vi "GPIB write rf ramp linear up for SG380.vi"(3 "calculate":bool, 5 "do it!":bool, 6 "debug":bool, 7 "time step (ms)":dbl=50.0 format="%.2f", 8 "Sweeps":T1(array[cluster])=[{"Enable MW"=FALSE, "MW End freq"="6810", "MW Tau (s)"="7", "MW Amplitude (dB)"="-3", "MW Comments"=""}, {"Enable MW"=FALSE, "MW End freq"="6820", "MW Tau (s)"="7", "MW Amplitude (dB)"="-5", "MW Comments"=""}, {"Enable MW"=FALSE, "MW End freq"="6830", "MW Tau (s)"="5", "MW Amplitude (dB)"="-5", "MW Comments"=""}, {"Enable MW"=FALSE, "MW End freq"="6832", "MW Tau (s)"="1", "MW Amplitude (dB)"="-7", "MW Comments"=""}, {"Enable MW"=FALSE, "MW End freq"="6833.22", "MW Tau (s)"="1", "MW Amplitude (dB)"="-8", "MW Comments"=""}], 9 "start freq (MHz)":string="6700.00", 10 "start time (sec)":string="1.000") -> (0 "start freq 2":dbl=6700.0, 1 "start time 2":dbl=1.0, 2 "calc'd time":dbl=1.0 format="%.3f", 4 "timing check":dbl=6.484375 format="%.3f")   [LabVIEW 2017]
uses:
  <vilib>/Utility/file.llb/Write Delimited Spreadsheet (DBL).vi
panel:
  out "Numeric":i32
  out "error out 3":errorcluster={"status"=TRUE, "code"=2, "source"="GPIB Write in rf ramp newest.vi"}
  in  "write":string="FREQ 6 MHz"
  in  "TEST":bool
  in  "GPIB address":string="27"
  out "error out 2":errorcluster={"status"=TRUE, "code"=7, "source"="GPIB Write in GPIB write rf ramp linear up for SG380.vi->host 1st.vi"}
  out "New sweeps array":dbl[][](array[numeric])
  out "error out":errorcluster
  out "XY Graph":cluster{"times":dbl[], "freqs":dbl[]}(graph)
  out "freqs":dbl[](array[numeric]) format="%.2f"
  out "times":dbl[](array[numeric])=[6700.0] format="%.2f"
  out "Path":path=path "C:/Debbie/experiment stuff/B231/13 Experiment Control/C code files/rf Ramp (2003 July 18)/rf ramp debug.txt"
  out "clock start":dbl=3608801724.173161 format="%.2f"
  out "freqs":dbl[](array[numeric])=[6700.0] format="%.2f"
  out "nramps":i32
  # "enable     f (MHz)           tau (sec)             ampl (dBm)                    notes"
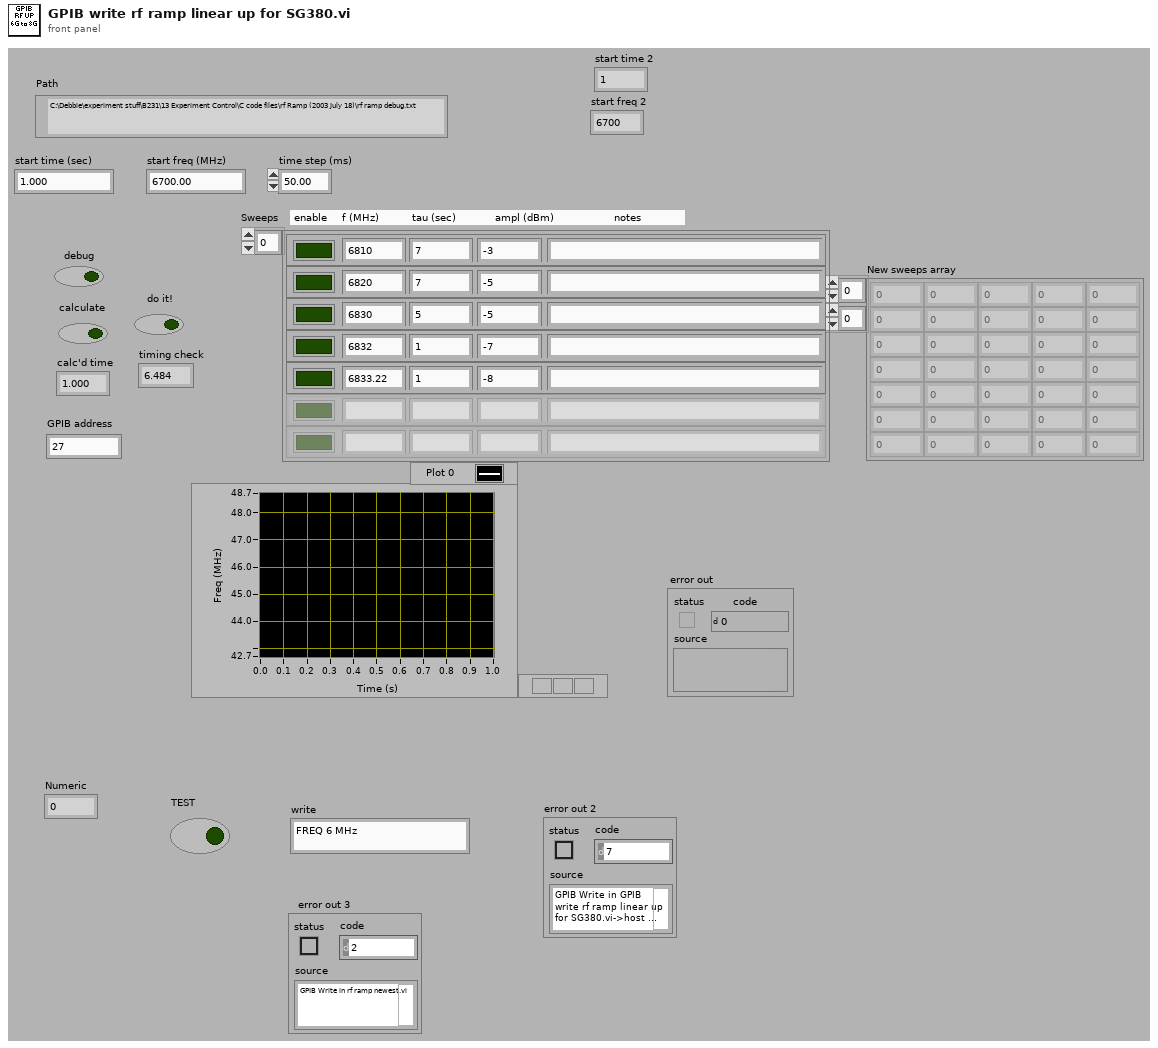
[diagram p1: front panel]
types:
  T1 = cluster{"Enable MW":bool, "MW End freq":string, "MW Tau (s)":string, "MW Amplitude (dB)":string, "MW Comments":string}[]
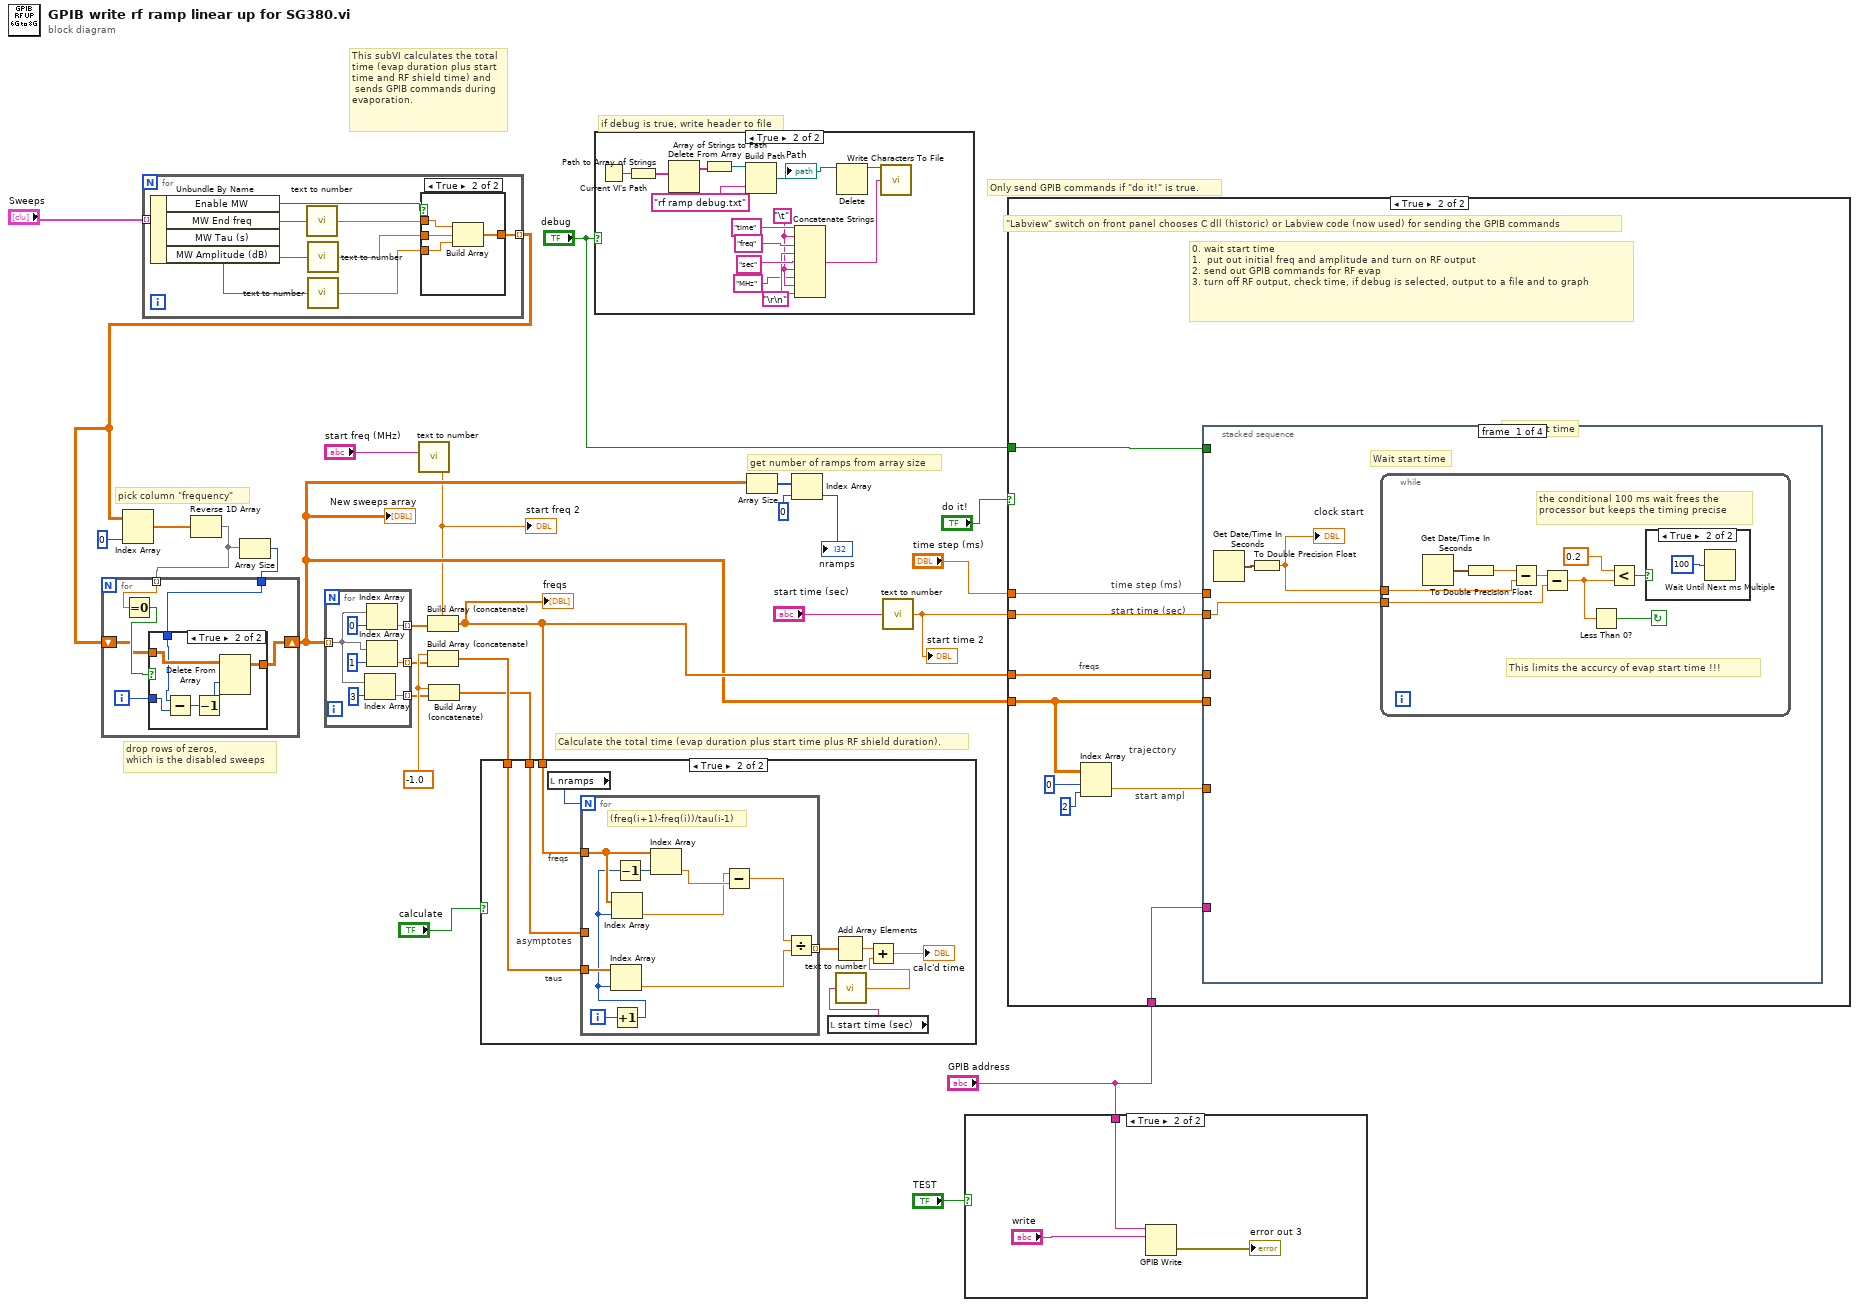
[diagram p0: block diagram]
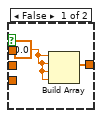
[diagram p4: hidden frame]
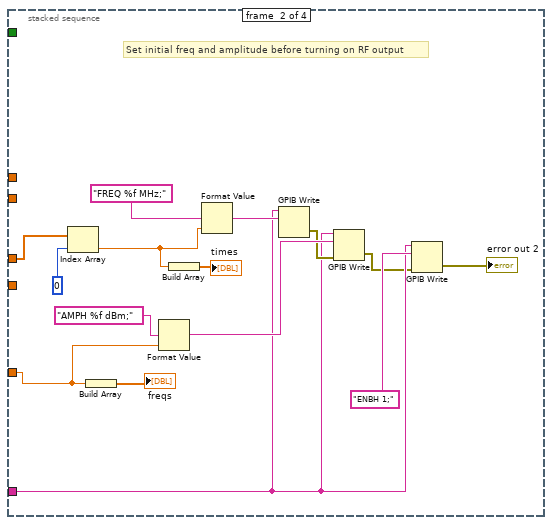
[diagram p7: hidden frame]
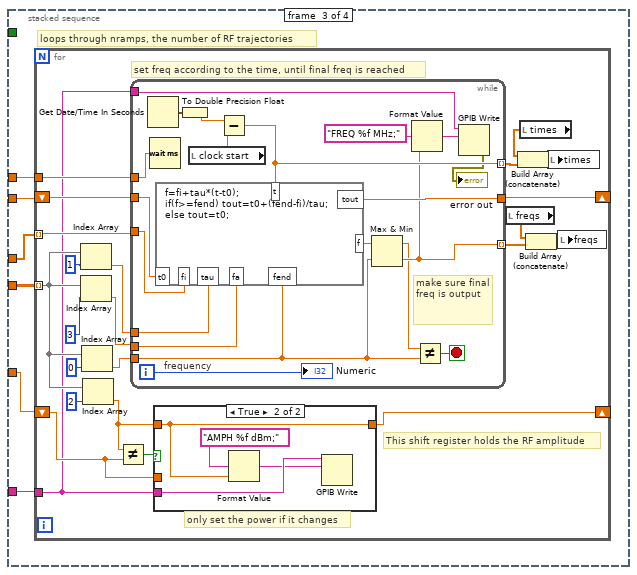
[diagram p8: hidden frame]
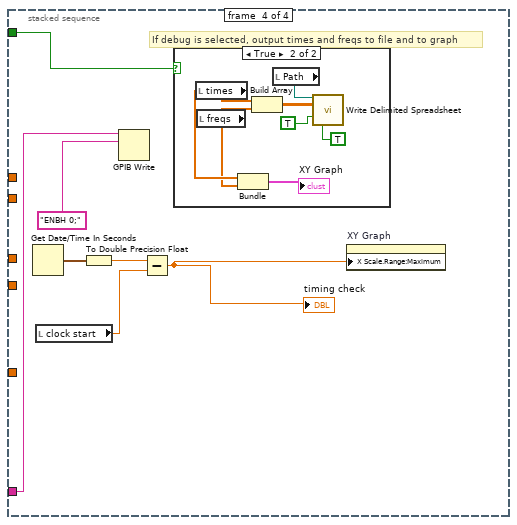
[diagram p10: hidden frame]
diagram:
  w18 = -1.0
  # "drop rows of zeros,\nwhich is the disabled sweeps"
  # "pick column \"frequency\""
  # "Only send GPIB commands if \"do it!\" is true."
  # "if debug is true, write header to file"
  # "This subVI calculates the total time (evap duration plus start time and RF shield time) and\n sends GPIB commands during evaporation."
  # "Calculate the total time (evap duration plus start time plus RF shield duration)."
  # "get number of ramps from array size"
  n1 = for {
    tunnel: "Sweeps" -> [w36] mode=indexing
    tunnel: [w34] -> w15 mode=indexing
    n2 = Unbundle By Name(w36) -> ("Enable MW"=w35:bool, "MW End freq"=w33:string, "MW Tau (s)"=w31:string, "MW Amplitude (dB)"=w30:string)
    n3 = call "text to number.vi"("text"=w33) -> ("number"=w32:dbl)
    n4 = call "text to number.vi"("text"=w31) -> ("number"=w29:dbl)
    n5 = call "text to number.vi"("text"=w30) -> ("number"=w28:dbl)
    n6 = case shown="True" w35 {
      tunnel: w32 -> [_ w42]
      tunnel: w29 -> [_ w41]
      tunnel: w28 -> [_ w40]
      tunnel: [w38 w39] -> w34
      frame False {
        w37 = 0.0 ("element")
        n7 = Build Array(w37, w37, w37, w37) -> (w38:dbl[])
      }
      frame True {
        n8 = Build Array(w42, w41, w40) -> (w39:dbl[])
      }
    }
  }
  n9 = Index Array(array=w15, index (col)=i8 0 ("Column #")) -> (element=w8:dbl[])  [unwired: 1 in]
  n10 = Reverse 1D Array(array=w8) -> (reversed array=w7:dbl[])
  n11 = Array Size(array=w7) -> (size(s)=w6:i32)
  n12 = for {
    tunnel: w7 -> [w48] mode=indexing
    shift-right: [w45] -> w9
    shift-left: w15 -> [w46]
    tunnel: w6 -> [w44]
    i -> [w43]
    n13 = Equal To 0?(x=w48) -> (x = 0?=w47:bool)
    n14 = case shown="True" w47 {
      tunnel: w46 -> [w49 w55]
      tunnel: w43 -> [_ w52]
      tunnel: [w49 w54] -> w45
      tunnel: w44 -> [_ w53]
      frame False {
      }
      frame True {
        n15 = Subtract(x=w53, y=w52) -> (x-y=w50:i32)
        n16 = Decrement(x=w50) -> (x-1=w51:i32)
        n17 = Delete From Array(array=w55, index (row)=w51) -> (array with subset deleted=w54:dbl[][])  [unwired: 2 in, 1 out]
      }
    }
  }
  "New sweeps array" <- w9
  n18 = for {
    tunnel: [w60] -> w12 mode=indexing
    tunnel: [w59] -> w11 mode=indexing
    tunnel: [w57] -> w10 mode=indexing
    tunnel: w9 -> [w56] mode=indexing
    n19 = Index Array(array=w56, index=3 ("Index")) -> (element=w57:dbl)
    n20 = Index Array(array=w56, index=0 ("Index")) -> (element=w60:dbl)
    n21 = Index Array(array=w56, index=1 ("Index")) -> (element=w59:dbl)
  }
  n22 = call "text to number.vi"("text"="start freq (MHz)") -> ("number"=w3:dbl)
  "start freq 2" <- w3
  n23 = Build Array (concatenate)(w3, w12) -> (w22:dbl[])
  "freqs" <- w22
  n24 = Build Array (concatenate)(w18, w11) -> (w21:dbl[])
  n25 = Build Array (concatenate)(w18, w10) -> (w20:dbl[])
  n26 = case shown="True" "calculate" {
    tunnel: w22 -> [_ w70]
    tunnel: w21 -> [_ w69]
    tunnel: w20 -> [_ w66]
    frame False {
    }
    frame True {
      # "taus"
      # "asymptotes"
      # "freqs"
      n27 = local read "nramps"() -> (w71:i32)
      n28 = for {
        N: w71 -> [_]
        tunnel: w70 -> [w79]
        tunnel: w69 -> [w81]
        tunnel: [w76] -> w68 mode=indexing
        tunnel: w66 -> [_]
        i -> [w78]
        # "(freq(i+1)-freq(i))/tau(i-1)"
        n29 = Increment(x=w78) -> (x+1=w77:i32)
        n30 = Index Array(array=w81, index=w77) -> (element=w75:dbl)
        n31 = Index Array(array=w79, index=w77) -> (element=w72:dbl)
        n32 = Decrement(x=w77) -> (x-1=w80:i32)
        n33 = Index Array(array=w79, index=w80) -> (element=w73:dbl)
        n34 = Subtract(x=w72, y=w73) -> (x-y=w74:dbl)
        n35 = Divide(x=w74, y=w75) -> (x/y=w76:dbl)
      }
      n36 = local read "start time (sec)"() -> (w64:string)
      n37 = Add Array Elements(numeric array=w68) -> (sum=w67:dbl)
      n38 = call "text to number.vi"("text"=w64) -> ("number"=w63:dbl)
      n39 = Add(x=w67, y=w63) -> (x+y=→"calc'd time":dbl)
    }
  }
  n40 = case shown="True" "debug" {
    frame False {
    }
    frame True {
      w87 = "\r\n"
      w85 = "\t"
      n41 = Current VI's Path() -> (path=w95:path)
      n42 = Path to Array of Strings(0:w95) -> (2:w94:string[])  [unwired: 1 out]
      n43 = Delete From Array(array=w94) -> (array with subset deleted=w93:string[])  [unwired: 2 in, 1 out]
      n44 = Array of Strings to Path(0:w93) -> (2:w92:path)  [unwired: 1 in]
      n45 = Build Path(base path=w92, name or relative path="rf ramp debug.txt") -> (appended path=w83:path)
      "Path" <- w83
      n46 = Concatenate Strings("time", w85, "freq" ("Substring"), w87, "sec" ("Substring"), w85, "MHz" ("Substring"), w85, w87) -> (w86:string)
      n47 = Delete(path (use dialog)=w83) -> (deleted path=w82:path)  [unwired: 4 in, 2 out]
      n48 = call <vilib>:"Write Characters To File.vi"("character string"=w86, "file path (dialog if empty)"=w82) -> ()  [unwired: 3 in, 1 out]
    }
  }
  n49 = Array Size(array=w9) -> (size(s)=w14:i32[])
  n50 = Index Array(array=w14, index=0 ("Index")) -> (element=→"nramps":i32)
  n51 = call "text to number.vi"("text"="start time (sec)") -> ("number"=w1:dbl)
  "start time 2" <- w1
  n52 = case shown="True" "TEST" {
    tunnel: "GPIB address" -> [_ w98]
    frame False {
    }
    frame True {
      n53 = GPIB Write(0:w98, 1:"write") -> (6:→"error out 3":errorcluster)  [unwired: 3 in, 1 out]
    }
  }
  n54 = case shown="True" "do it!" {
    tunnel: w1 -> [_ w107]
    tunnel: "time step (ms)" -> [_ w106]
    tunnel: w22 -> [_ w105]
    tunnel: "debug" -> [_ w104]
    tunnel: w9 -> [_ w100]
    tunnel: "GPIB address" -> [_ w99]
    frame False {
    }
    frame True {
      # "freqs"
      # "trajectory"
      # "start ampl"
      # "time step (ms)"
      # "0. wait start time\n1.  put out initial freq and amplitude and turn on RF output\n2. send out GPIB commands for RF evap\n3. turn off RF output, check time, if debug is selected, output to a file and to graph"
      # "start time (sec)"
      # "\"Labview\" switch on front panel chooses C dll (historic) or Labview code (now used) for sending the GPIB commands"
      n55 = Index Array(array=w100, index (row)=0 ("Index"), index (col)=2 ("Disabled Index (col)")) -> (element=w102:dbl)
      n56 = stacked-sequence {
        tunnel: w107 -> [w110 _ w140 _]
        tunnel: w106 -> [_ _ w141 _]
        tunnel: w105 -> [_ w134 w139 _]
        tunnel: w102 -> [_ w129 w138 _]
        tunnel: w104 -> [_ _ _ w194]
        tunnel: w100 -> [_ _ w137 _]
        tunnel: w99 -> [_ w122 w136 w191]
        frame #0 {
          # "Wait start time"
          # "wait start time"
          n57 = Get Date/Time In Seconds() -> (seconds since 1Jan1904=w109:timestamp)
          n58 = To Double Precision Float(number=w109) -> (double precision float=w108:dbl)
          "clock start" <- w108
          n59 = while {
            tunnel: w108 -> [w112]
            tunnel: w110 -> [w118]
            stop <- w113 continue-if-true
            # "This limits the accurcy of evap start time !!!"
            # "the conditional 100 ms wait frees the processor but keeps the timing precise"
            n60 = Get Date/Time In Seconds() -> (seconds since 1Jan1904=w111:timestamp)
            n61 = To Double Precision Float(number=w111) -> (double precision float=w119:dbl)
            n62 = Subtract(x=w119, y=w112) -> (x-y=w115:dbl)
            n63 = Subtract(x=w115, y=w118) -> (x-y=w114:dbl)
            n64 = Less Than 0?(x=w114) -> (x < 0?=w113:bool)
            n65 = Less?(x=0.2 ("y"), y=w114) -> (x < y?=w116:bool)
            n66 = case shown="True" w116 {
              frame False {
              }
              frame True {
                n67 = Wait Until Next ms Multiple(millisecond multiple=u32 100) -> ()  [unwired: 1 out]
              }
            }
          }
        }
        frame #1 {
          # "Set initial freq and amplitude before turning on RF output"
          n68 = Index Array(array=w134, index=0 ("Index")) -> (element=w130:dbl)
          n69 = Build Array(w129) -> (→"freqs":dbl[])
          n70 = Format Value(format string="AMPH %f dBm;", value (0)=w129) -> (output string=w126:string)  [unwired: 1 in]
          n71 = Build Array(w130) -> (→"times":dbl[])
          n72 = Format Value(format string="FREQ %f MHz;", value (0)=w130) -> (output string=w127:string)  [unwired: 1 in]
          n73 = GPIB Write(0:w122, 1:w127) -> (6:w125:errorcluster)  [unwired: 3 in, 1 out]
          n74 = GPIB Write(0:w122, 1:w126, 3:w125) -> (6:w121:errorcluster)  [unwired: 2 in, 1 out]
          n75 = GPIB Write(0:w122, 1:"ENBH 1;" ("data"), 3:w121) -> (6:→"error out 2":errorcluster)  [unwired: 2 in, 1 out]
        }
        frame #2 {
          # "loops through nramps, the number of RF trajectories"
          n76 = for {
            tunnel: w141 -> [w164]
            shift-right: [w156] -> _
            shift-left: w140 -> [w159]
            tunnel: w139 -> [w158] mode=indexing
            shift-right: [w143] -> _
            shift-left: w138 -> [w144]
            tunnel: w137 -> [w146] mode=indexing
            tunnel: w136 -> [w142]
            # "This shift register holds the RF amplitude"
            # "set freq according to the time, until final freq is reached"
            # "only set the power if it changes"
            n77 = Index Array(array=w146, index=1 ("Index")) -> (element=w160:dbl)
            n78 = Index Array(array=w146, index=3 ("Index")) -> (element=w155:dbl)
            n79 = Index Array(array=w146, index=0 ("Index")) -> (element=w154:dbl)
            n80 = Index Array(array=w146, index=2 ("Index")) -> (element=w145:dbl)
            n81 = Not Equal?(x=w145, y=w144) -> (x != y?=w153:bool)
            n82 = while {
              tunnel: [w176] -> w152 mode=indexing
              tunnel: [w169] -> w149 mode=indexing
              tunnel: [w179] -> w156
              tunnel: w158 -> [w181]
              tunnel: w159 -> [w180]
              tunnel: w155 -> [w172]
              tunnel: w160 -> [w173]
              tunnel: w154 -> [w171]
              tunnel: w164 -> [w183]
              tunnel: w142 -> [w167]
              i -> [w170]
              stop <- w182 stop-if-true
              # "make sure final freq is output"
              # "frequency"
              n83 = Get Date/Time In Seconds() -> (seconds since 1Jan1904=w174:timestamp)
              n84 = Wait (ms)(milliseconds to wait=w183) -> ()  [unwired: 1 out]
              n85 = To Double Precision Float(number=w174) -> (double precision float=w184:dbl)
              n86 = local read "clock start"() -> (w178:dbl)
              n87 = Subtract(x=w184, y=w178) -> (x-y=w176:dbl)
              n88 = formula code="f=fi+tau*(t-t0);\nif(f>=fend) tout=t0+(fend-fi)/tau;\nelse tout=t0;"("fi"=w181, "tau"=w173, "fa"=w172, "t0"=w180, "t"=w176, "fend"=w171) -> ("f"=w175:dbl, "tout"=w179:dbl)
              n89 = Max & Min(x=w175, y=w171) -> (max(x,y)=w168:dbl, min(x,y)=w169:dbl)
              n90 = Format Value(format string="FREQ %f MHz;", value (0)=w169) -> (output string=w166:string)  [unwired: 1 in]
              n91 = Not Equal?(x=w168, y=w171) -> (x != y?=w182:bool)
              n92 = GPIB Write(0:w167, 1:w166) -> (6:→"error out":errorcluster)  [unwired: 3 in, 1 out]
              "Numeric" <- w170
            }
            n93 = case shown="True" w153 {
              tunnel: w145 -> [w185 w188]
              tunnel: [w185 w188] -> w143
              tunnel: w144 -> [_ _]
              tunnel: w142 -> [_ w187]
              frame False {
              }
              frame True {
                n94 = Format Value(format string="AMPH %f dBm;", value (0)=w188) -> (output string=w186:string)  [unwired: 1 in]
                n95 = GPIB Write(0:w187, 1:w186) -> ()  [unwired: 3 in, 2 out]
              }
            }
            n96 = local read "freqs"() -> (w147:dbl[])
            n97 = local read "times"() -> (w151:dbl[])
            n98 = Build Array (concatenate)(w151, w152) -> (w150:dbl[])
            n99 = Build Array (concatenate)(w147, w149) -> (w148:dbl[])
            n100 = local write "times"(w150) -> ()
            n101 = local write "freqs"(w148) -> ()
          }
        }
        frame #3 {
          # "If debug is selected, output times and freqs to file and to graph"
          n102 = Get Date/Time In Seconds() -> (seconds since 1Jan1904=w193:timestamp)
          n103 = local read "clock start"() -> (w195:dbl)
          n104 = To Double Precision Float(number=w193) -> (double precision float=w196:dbl)
          n105 = GPIB Write(0:w191, 1:"ENBH 0;" ("data")) -> ()  [unwired: 3 in, 2 out]
          n106 = Subtract(x=w196, y=w195) -> (x-y=w190:dbl)
          "timing check" <- w190
          n107 = case shown="True" w194 {
            frame False {
            }
            frame True {
              n108 = local read "times"() -> (w202:dbl[])
              n109 = local read "freqs"() -> (w198:dbl[])
              n110 = Bundle("times"=w202, "freqs"=w198) -> (→"XY Graph":cluster{"times":dbl[], "freqs":dbl[]})  [unwired: 1 in]
              n111 = Build Array(w202, w198) -> (w199:dbl[][])
              n112 = local read "Path"() -> (w203:path)
              n113 = call-poly <vilib>:"Write Delimited Spreadsheet.vi"("file path (dialog if empty)"=w203, "2D data"=w199, "append to file? (new file:F)"=TRUE, "transpose? (no:F)"=TRUE) -> ()  [unwired: 10 in, 2 out]
            }
          }
          n114 = property on="XY Graph" class="XYGraph (strict)"("X Scale.Range:Maximum"=w190) -> ()  [unwired: 2 in, 2 out]
        }
      }
    }
  }
